vi "main.vi"() -> ()   [LabVIEW 2010]
uses:
  common/clusters/plugin_specification.ctl
  item_creation_flags_cluster.ctl
  common/classes/GenericComponent/GenericComponent/GenericComponent.lvclass
panel:
  in  "Run method?":bool
  in  "Settings file?":bool
  in  "Terminate method?":bool
  in  "Initialize method?":bool
  in  "Subcomponents?":bool
  in  "Configuration file?":bool
  in  "stopButton":bool
  in  "createButton":bool
  in  "parent component path":path
  in  "postfix":string
  in  "your initials":string
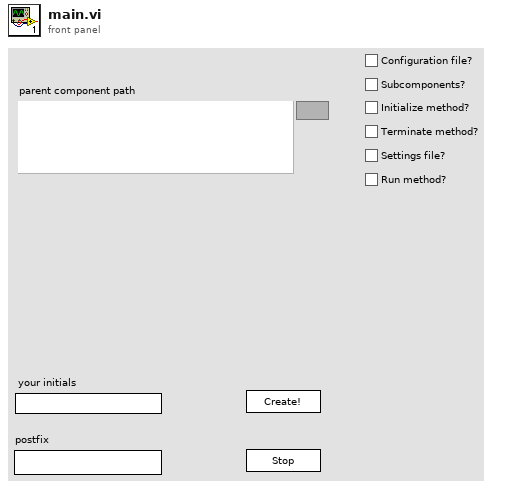
[diagram p1: front panel]
types:
  T1 = typedef "plugin_specification.ctl" = cluster{"class path":string, "configuration":string, "label":string, "settings name":string}
  T2 = typedef "item_creation_flags_cluster.ctl" = cluster{"configuration file?":bool, "subcomponents?":bool, "initialize method?":bool, "terminate method?":bool, "settings file":bool, "run method?":bool}
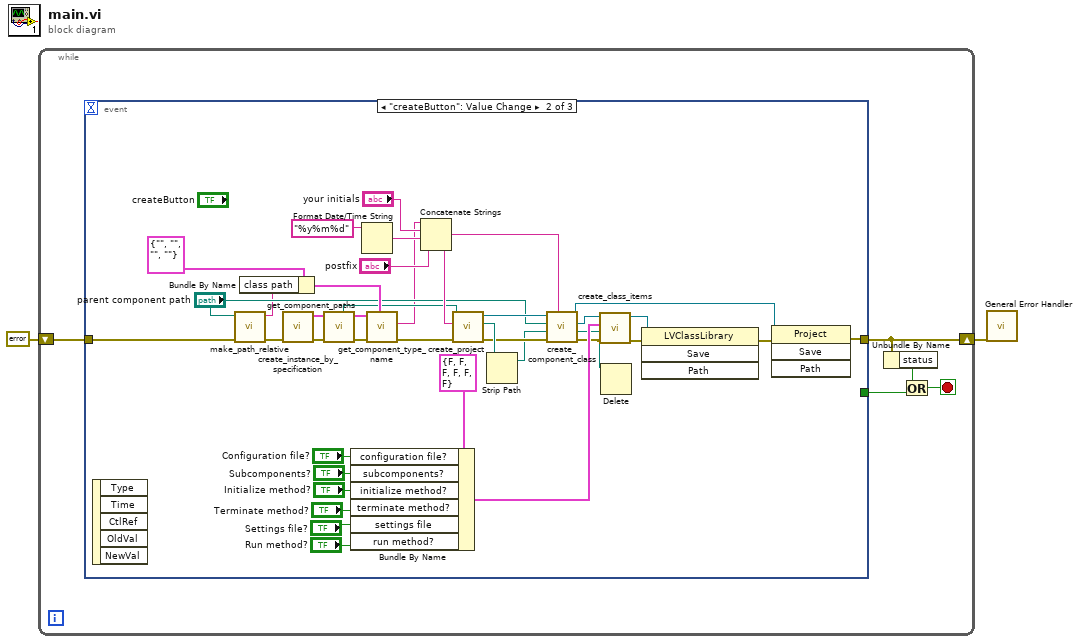
[diagram p0: block diagram]
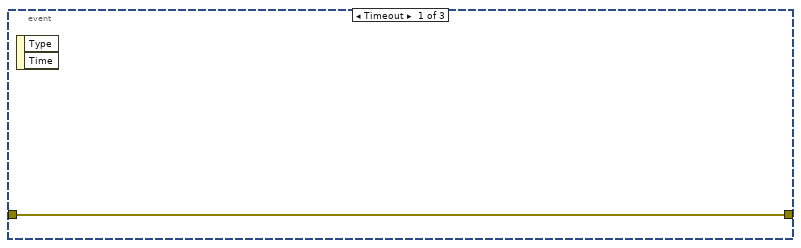
[diagram p2: hidden frame]
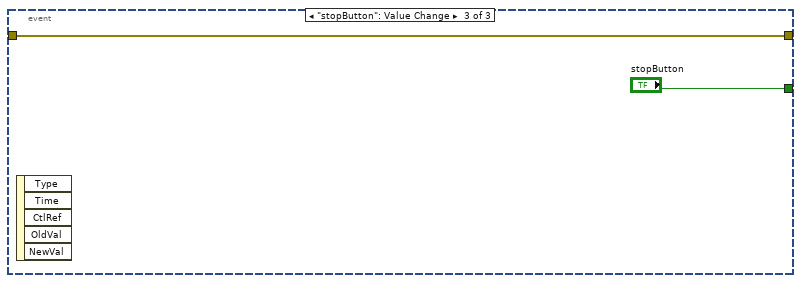
[diagram p3: hidden frame]
diagram:
  n1 = while {
    shift-right: [w6] -> w1
    shift-left: errorcluster {"status"=FALSE, "code"=0, "source"=""} ("error out") -> [w7]
    stop <- w4 stop-if-true
    n2 = event shown="[1] \"createButton\": Value Change" {
      selector: _ -> [_ _ _]
      dyn-events: _ -> [_ _ _]
      timeout: _ -> [_ _ _]
      tunnel: [w8 w37 w48] -> w6
      tunnel: w7 -> [w8 w21 w48]
      tunnel: [_ _ "stopButton"] -> w3
      event Timeout {
        n3 = event-data() -> ()  [unwired: 1 in, 2 out]
      }
      event "createButton": Value Change {
        n4 = event-data() -> ()  [unwired: 1 in, 5 out]
        n5 = call "make_path_relative.vi"("error in (no error)"=w21, "absolute path"="parent component path") -> ("error out"=w22:errorcluster, "relative path"=w29:string)  [unwired: 8 in]
        n6 = Bundle By Name(cluster=T1 {"class path"="", "configuration"="", "label"="", "settings name"=""} ("component specification"), "class path"=w29) -> (w31:T1)
        n7 = call "create_instance_by_specification.vi"("error in (no error)"=w22, "component specification"=w31) -> ("error out"=w27:errorcluster, "GenericPlugin out"=w28:refnum<class "GenericComponent.lvclass">)  [unwired: 7 in, 1 out]
        n8 = call-dynamic "get_component_paths.vi"("error in (no error)"=w27, "GenericComponent in"=w28) -> ("error out"=w26:errorcluster, "GenericComponent out"=w25:refnum<class "GenericComponent.lvclass">, "component type directory"=w24:path)  [unwired: 4 in, 3 out]
        n9 = Bundle By Name(cluster=T2 {"configuration file?"=FALSE, "subcomponents?"=FALSE, "initialize method?"=FALSE, "terminate method?"=FALSE, "settings file"=FALSE, "run method?"=FALSE} ("item creation flags"), "configuration file?"="Configuration file?", "subcomponents?"="Subcomponents?", "initialize method?"="Initialize method?", "terminate method?"="Terminate method?", "settings file"="Settings file?", "run method?"="Run method?") -> (w19:T2)
        n10 = Format Date/Time String(time format string (%c)="%y%m%d") -> (date/time string=w40:string)  [unwired: 2 in]
        n11 = call-dynamic "get_component_type_name.vi"("error in (no error)"=w26, "GenericPlugin in"=w25) -> ("error out"=w20:errorcluster, "component type"=w23:string)  [unwired: 7 in, 1 out]
        n12 = Concatenate Strings(w23, "your initials", w40, "postfix") -> (w44:string)
        n13 = call "create_project.vi"("error in (no error)"=w20, "component name"=w44, "target folder path"=w24) -> ("error out"=w43:errorcluster, "component project path"=w45:path, "project reference out"=w42:refnum<vi>)  [unwired: 6 in]
        n14 = Strip Path(path=w45) -> (stripped path=w11:path)  [unwired: 1 out]
        n15 = call "create_component_class.vi"("component name"=w44, "error in (no error)"=w43, "component project folder path"=w11, "parent component class path"="parent component path", "project reference in"=w42) -> ("error out"=w18:errorcluster, "new component template path"=w10:path, "new class reference out"=w15:refnum<vi>, "project reference out"=w16:refnum<vi>)  [unwired: 3 in]
        n16 = call "create_class_items.vi"("error in"=w18, "item creation flags"=w19, "new class reference in"=w15) -> ("error out"=w17:errorcluster, "new class reference out"=w14:refnum<vi>)  [unwired: 7 in]
        n17 = Delete(path (use dialog)=w10) -> ()  [unwired: 4 in, 3 out]
        n18 = invoke class="LVClassLibrary" method="Save"(reference=w14, error in=w17) -> (error out=w46:errorcluster)  [unwired: 2 in, 3 out]
        n19 = invoke class="Project" method="Save"(reference=w16, error in=w46) -> (error out=w37:errorcluster)  [unwired: 2 in, 3 out]
      }
      event "stopButton": Value Change {
        n20 = event-data() -> ()  [unwired: 1 in, 5 out]
      }
    }
    n21 = Unbundle By Name(w6) -> ("status"=w5:bool)
    n22 = Or(x=w5, y=w3) -> (x .or. y?=w4:bool)
  }
  n23 = call <vilib>:"General Error Handler.vi"("error in (no error)"=w1) -> ()  [unwired: 10 in, 5 out]
